vi "FFT - Auto Power Spectrums.vi"(0 "reference in":refnum<class "GSwFormDSP.lvclass">, 5 "error in (no error)":errorcluster) -> (13 "Nb Averages":i32[](array[numeric]), 14 "reference out":refnum<class "GSwFormDSP.lvclass">, 19 "error out":errorcluster)   [LabVIEW 2020, in "GSwFormDSP.lvclass"]
uses:
  GSwFormDSP.lvclass
  <vilib>/Analysis/0measdsp.llb/Scaled Time Domain Window (DBL).vi
  <vilib>/Analysis/NI_AALPro.lvlib
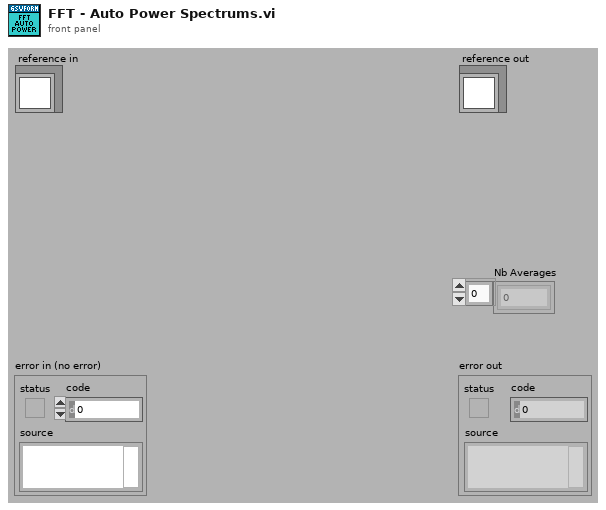
[diagram p1: front panel]
types:
  T1 = typedef "GSwFormDSP.lvclass/ObjectAttributesRef.ctl" = refnum<data-value>
  T2 = typedef "GSwFormDSP.lvclass/ObjectAttributes.ctl" = cluster{"Wform Ref":refnum<data-value>, "Nb Signals":i32, "Spectral Function Parameters":T3, "FFT":waveform(cdb)[], "Nb FFT":i32, "Nb Averages":i32[], "Reference Indexes":i32[], "Response Indexes":i32[], "Coherence":waveform(dbl)[], "TDF Parameters":T5, "DAQ":cluster{"Duration (sec)":dbl, "Buffer Size (Samples)":i32, "Offset (Samples)":i32}, "Filter Impulse Response (TDF)":waveform(dbl), "Sound Playback":T6}
  T3 = typedef "GSwFormDSP.lvclass/Spectral Parameters.ctl" = cluster{"Frequency resolution (Hz)":dbl, "Overlap":dbl, "Window":T4}
  T4 = typedef "NI_AALPro.lvlib/windowTd.ctl" = u32
  T5 = typedef "GSwFormDSP.lvclass/TDF Parameters.ctl" = cluster{"Filter":enum32{"Lowpass", "Highpass", "Bandpass", "Bandstop"}, "Type:":enum16{"Butterworth", "Chebyshev", "Inv Chebyshev", "Elliptic", "Bessel"}, "LP cutoff freq":dbl, "HP cutoff freq":dbl, "Order":i32, "passband ripple (dB)":dbl, "stopband attenuation (dB)":dbl, "Phaseless Filter":bool, "Include Fade IN and OUT":bool}
  T6 = typedef "GSwFormDSP.lvclass/Sound Playback.ctl" = cluster{"Timer start (ms)":u32, "task ID":T7, "Cursor Init Location (s)":dbl, "SC Volume":dbl}
  T7 = typedef "Sound Output Task ID.ctl" = u32
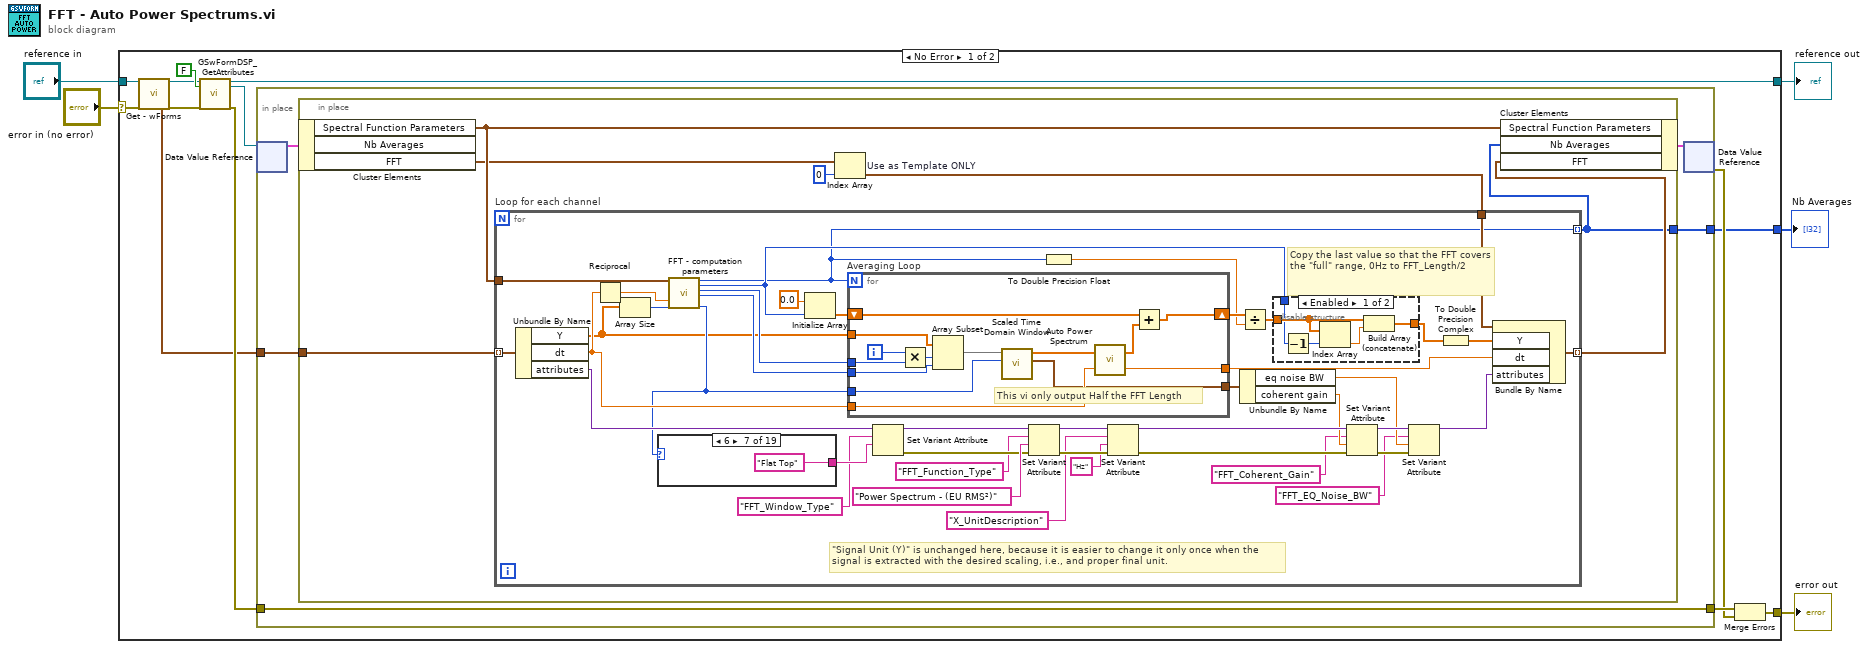
[diagram p0: block diagram]
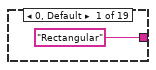
[diagram p3: hidden frame]
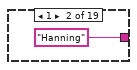
[diagram p4: hidden frame]
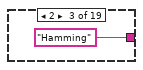
[diagram p5: hidden frame]
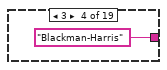
[diagram p6: hidden frame]
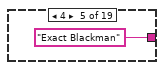
[diagram p7: hidden frame]
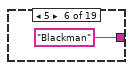
[diagram p8: hidden frame]
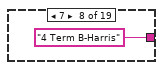
[diagram p9: hidden frame]
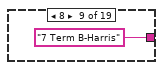
[diagram p10: hidden frame]
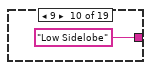
[diagram p11: hidden frame]
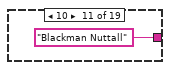
[diagram p12: hidden frame]
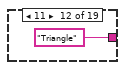
[diagram p13: hidden frame]
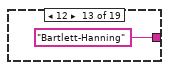
[diagram p14: hidden frame]
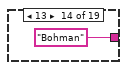
[diagram p15: hidden frame]
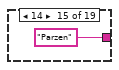
[diagram p16: hidden frame]
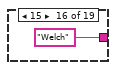
[diagram p17: hidden frame]
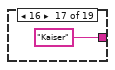
[diagram p18: hidden frame]
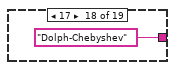
[diagram p19: hidden frame]
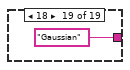
[diagram p20: hidden frame]
diagram:
  n1 = case shown="No Error" "error in (no error)" {
    selector: "error in (no error)" -> [w9 w114]
    tunnel: [w18 w114] -> w4
    tunnel: [w14 w113] -> w2
    tunnel: "reference in" -> [w10 w113]
    tunnel: [w11 i32[] []] -> w1
    frame No Error {
      n2 = call-dynamic "Get - wForms.vi"("reference in"=w10, "error in (no error)"=w9) -> ("wForms"=w6:waveform(dbl)[], "reference out"=w7:refnum<class "GSwFormDSP.lvclass">, "error out"=w8:errorcluster)  [unwired: 14 in, 1 out]
      n3 = call "GSwFormDSP_GetAttributes.vi"("reference in"=w7, "return data? (T)"=FALSE, "error in (no error)"=w8) -> ("reference out"=w14:refnum<class "GSwFormDSP.lvclass">, "attributes ref"=w13:T1, "error out"=w15:errorcluster)  [unwired: 13 in, 1 out]
      n4 = in-place {
        in-place-border: w15 -> [w21]
        in-place-border: [w21] -> w17
        in-place-border: [w20] -> w11
        in-place-border: w6 -> [w19]
        n5 = in-place-dvr #1(w13) -> (w22:T2)  [unwired: 1 out]
        n6 = in-place {
          in-place-border: [w25] -> w20
          in-place-border: w19 -> [w24]
          n7 = in-place-cluster #2(w22) -> ("Spectral Function Parameters"=w29:T3, "FFT"=w28:waveform(cdb)[])  [unwired: 1 out]
          n8 = Index Array "Use as Template ONLY"(array=w28, index=0) -> (element=w26:waveform(cdb))
          n9 = for "Loop for each channel" {
            tunnel: w24 -> [w32] mode=indexing
            tunnel: [w72] -> w30 mode=indexing
            tunnel: w29 -> [w71]
            tunnel: w26 -> [w35]
            tunnel: [w31] -> w25 mode=indexing
            # "Copy the last value so that the FFT covers the \"full\" range, 0Hz to FFT_Length/2"
            # "\"Signal Unit (Y)\" is unchanged here, because it is easier to change it only once when the signal is extracted with the desired scaling, i.e., and proper final unit."
            n10 = Unbundle By Name(w32) -> ("Y"=w33:dbl[], "dt"=w62:dbl, "attributes"=w61:variant)
            n11 = Reciprocal(x=w62) -> (1/x=w63:dbl)
            n12 = Array Size(array=w33) -> (size(s)=w64:i32)
            n13 = call "FFT - computation parameters.vi"("Spectral Function Parameters"=w71, "Fs"=w63, "Time vector length (samples)"=w64) -> ("Nb Averages"=w31:i32, "FFT Length/2"=w37:i32, "FFT Length - Overlap"=w65:i32, "FFT Length"=w40:i32, "window"=w36:T4)  [unwired: 11 in, 1 out]
            n14 = case shown="6" w36 {
              tunnel: ["Rectangular" ("Abscissa.Unit (X)") "Hanning" ("Abscissa.Unit (X)") "Hamming" ("Abscissa.Unit (X)") "Blackman-Harris" ("Abscissa.Unit (X)") "Exact Blackman" ("Abscissa.Unit (X)") "Blackman" ("Abscissa.Unit (X)") "Flat Top" ("Abscissa.Unit (X)") "4 Term B-Harris" ("Abscissa.Unit (X)") "7 Term B-Harris" ("Abscissa.Unit (X)") "Low Sidelobe" ("Abscissa.Unit (X)") "Blackman Nuttall" ("Abscissa.Unit (X)") "Triangle" ("Abscissa.Unit (X)") "Bartlett-Hanning" ("Abscissa.Unit (X)") "Bohman" ("Abscissa.Unit (X)") "Parzen" ("Abscissa.Unit (X)") "Welch" ("Abscissa.Unit (X)") "Kaiser" ("Abscissa.Unit (X)") "Dolph-Chebyshev" ("Abscissa.Unit (X)") "Gaussian" ("Abscissa.Unit (X)")] -> w59
              frame 0, Default {
              }
              frame 1 {
              }
              frame 2 {
              }
              frame 3 {
              }
              frame 4 {
              }
              frame 5 {
              }
              frame 6 {
              }
              frame 7 {
              }
              frame 8 {
              }
              frame 9 {
              }
              frame 10 {
              }
              frame 11 {
              }
              frame 12 {
              }
              frame 13 {
              }
              frame 14 {
              }
              frame 15 {
              }
              frame 16 {
              }
              frame 17 {
              }
              frame 18 {
              }
            }
            n15 = Initialize Array(0.0, w37) -> (w69:dbl[])
            n16 = for "Averaging Loop" {
              N: w31 -> [_]
              shift-right: [w101] -> w68
              shift-left: w69 -> [w103]
              tunnel: w65 -> [w108]
              tunnel: w40 -> [w107]
              tunnel: w33 -> [w106]
              tunnel: w62 -> [w102]
              tunnel: [w100] -> w60
              tunnel: [w99] -> w66
              tunnel: w36 -> [w98]
              i -> [w109]
              # "This vi only output Half the FFT Length"
              n17 = Multiply(x=w109, y=w108) -> (x*y=w110:i32)
              n18 = Array Subset(array=w106, index=w110, length=w107) -> (w105:dbl[])
              n19 = call-poly <vilib>:"Scaled Time Domain Window.vi"("window"=w98, "X"=w105) -> ("window properties"=w99:cluster{"eq noise BW":dbl, "coherent gain":dbl}, "Windowed X"=w111:dbl[])  [unwired: 1 in, 7 out]
              n20 = call <vilib>:"Auto Power Spectrum.vi"("dt"=w102, "Signal (V)"=w111) -> ("df"=w100:dbl, "Power Spectrum (V^2 rms)"=w104:dbl[])
              n21 = Add(x=w103, y=w104) -> (x+y=w101:dbl[])
            }
            n22 = Set Variant Attribute(Variant=w61, name="FFT_Window_Type" ("Att - Window Type"), value=w59) -> (Variant out=w58:variant, error out=w56:errorcluster)  [unwired: 1 in, 1 out]
            n23 = Set Variant Attribute(Variant=w58, name="FFT_Function_Type" ("Att - Function Type"), value="Power Spectrum - (EU RMS²)" ("Ordinate.Function Description.Function Type"), error in=w56) -> (Variant out=w55:variant, error out=w54:errorcluster)  [unwired: 1 out]
            n24 = To Double Precision Float(number=w31) -> (double precision float=w67:dbl)
            n25 = Set Variant Attribute(Variant=w55, name="X_UnitDescription" ("X unit"), value="Hz" ("Abscissa.Unit (X)"), error in=w54) -> (Variant out=w52:variant, error out=w51:errorcluster)  [unwired: 1 out]
            n26 = Divide(x=w68, y=w67) -> (x/y=w38:dbl[])
            n27 = Unbundle By Name(w66) -> ("eq noise BW"=w47:dbl, "coherent gain"=w50:dbl)
            n28 = disable-structure shown="Enabled" {
              disable-tunnel: [w76 w78] -> w39
              disable-tunnel: w38 -> [w75 w78]
              disable-tunnel: w37 -> [w74 _]
              frame Enabled {
                n29 = Decrement(x=w74) -> (x-1=w73:i32)
                n30 = Index Array(array=w75, index=w73) -> (element=w77:dbl)
                n31 = Build Array (concatenate)(w75, w77) -> (w76:dbl[])
              }
              frame Disabled {
              }
            }
            n32 = Set Variant Attribute(Variant=w52, name="FFT_Coherent_Gain" ("Coherent Gain (DBL)"), value=w50, error in=w51) -> (Variant out=w48:variant, error out=w49:errorcluster)  [unwired: 1 out]
            n33 = Set Variant Attribute(Variant=w48, name="FFT_EQ_Noise_BW" ("EQ noise BW (DBL)"), value=w47, error in=w49) -> (Variant out=w46:variant)  [unwired: 2 out]
            n34 = To Double Precision Complex(1:w39) -> (0:w34:cdb[])
            n35 = Bundle By Name(cluster=w35, "Y"=w34, "dt"=w60, "attributes"=w46) -> (w72:waveform(cdb))
          }
          n36 = in-place-cluster #2("Spectral Function Parameters"=w29, "Nb Averages"=w25, "FFT"=w30) -> (w23:T2)
        }
        n37 = in-place-dvr #1(w23) -> (w12:errorcluster)  [unwired: 1 out]
      }
      n38 = Merge Errors(w17, w12) -> (w18:errorcluster)
    }
    frame Error {
    }
  }
  "error out" <- w4
  "reference out" <- w2
  "Nb Averages" <- w1
